vi "remove_tilt_from_displacement_vectors.vi"(1 "Array 2":cluster{dbl, dbl}[][](array[cluster]), 2 "Array 3":bool[][](array[boolean])) -> (0 "Array":cluster{dbl, dbl}[][](array[cluster]))   [LabVIEW 2010]
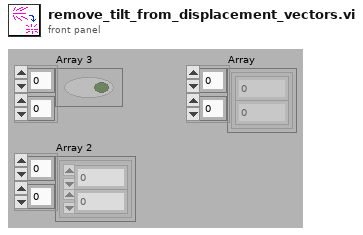
[diagram p1: front panel]
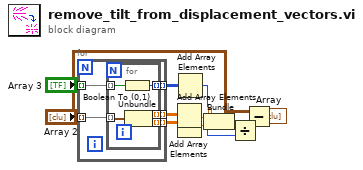
[diagram p0: block diagram]
diagram:
  n1 = for {
    tunnel: "Array 2" -> [w15] mode=indexing
    tunnel: "Array 3" -> [w16] mode=indexing
    tunnel: [w14] -> w2 mode=indexing
    tunnel: [w13] -> w3 mode=indexing
    tunnel: [w12] -> w4 mode=indexing
    n2 = for {
      tunnel: w16 -> [w20] mode=indexing
      tunnel: w15 -> [w21] mode=indexing
      tunnel: [w19] -> w14 mode=indexing
      tunnel: [w18] -> w13 mode=indexing
      tunnel: [w17] -> w12 mode=indexing
      n3 = Boolean To (0,1)(Boolean=w20) -> (0, 1=w19:i16)
      n4 = Unbundle(w21) -> (w17:dbl, w18:dbl)
    }
  }
  n5 = Add Array Elements(numeric array=w4) -> (sum=w7:dbl)
  n6 = Add Array Elements(numeric array=w3) -> (sum=w6:dbl)
  n7 = Add Array Elements(numeric array=w2) -> (sum=w5:i16)
  n8 = Bundle(w7, w6) -> (w8:cluster{dbl, dbl})  [unwired: 1 out]
  n9 = Divide(x=w8, y=w5) -> (x/y=w9:cluster{dbl, dbl})
  n10 = Subtract(x="Array 2", y=w9) -> (x-y=→"Array":cluster{dbl, dbl}[][])
